vi "Run.vi"(8 "error in (no error)":errorcluster, 11 "socket PUB in":refnum<class "socket PUB.lvclass">) -> (0 "error out":errorcluster, 3 "socket PUB out":refnum<class "socket PUB.lvclass">)   [LabVIEW 2018, in "socket PUB.lvclass"]
uses:
  socket PUB.lvclass
  C:/Users/devstaff/sparc4/s4gui/Versao ZeroMQ REQ-REP/SPARC4_GUI -v1.0.8 - com pacote communication manager/communication-manager/Socket/Socket.lvclass
  State Machine/CM_State Machine.lvclass
  Socket/Socket.lvclass
  RxTx/CM_RxTx.lvclass
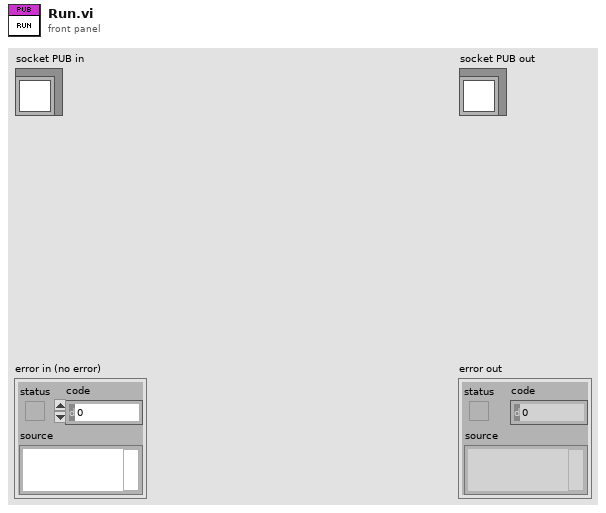
[diagram p1: front panel]
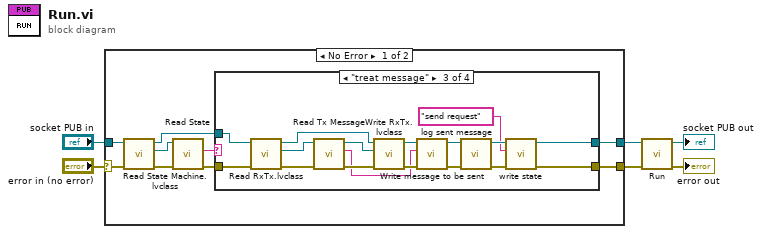
[diagram p0: block diagram]
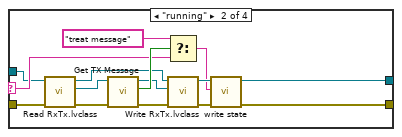
[diagram p3: hidden frame]
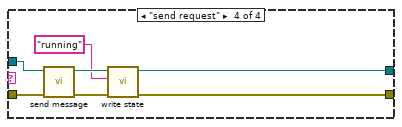
[diagram p4: hidden frame]
diagram:
  n1 = case shown="No Error" "error in (no error)" {
    selector: "error in (no error)" -> [w11 w57]
    tunnel: "socket PUB in" -> [w9 w58]
    tunnel: [w7 w58] -> w4
    tunnel: [w10 w57] -> w1
    frame No Error {
      n2 = call-dynamic "Read State Machine.lvclass.vi"("error in (no error)"=w11, "Socket in"=w9) -> ("error out"=w13:errorcluster, "State Machine.lvclass"=w15:refnum<class "CM_State Machine.lvclass">, "Socket out"=w8:refnum<class "socket PUB.lvclass">)  [unwired: 7 in]
      n3 = call-dynamic "Read State.vi"("error in (no error)"=w13, "State Machine in"=w15) -> ("error out"=w12:errorcluster, "State"=w14:string)  [unwired: 7 in, 1 out]
      n4 = case shown="\"treat message\"" w14 {
        selector: w14 -> [_ w31 _ _]
        tunnel: w8 -> [w17 w24 w42 w56]
        tunnel: [w17 w21 w34 w53] -> w7
        tunnel: [w16 w20 w33 w52] -> w10
        tunnel: w12 -> [w16 w29 w41 w55]
        frame Default {
        }
        frame "running" {
          n5 = call-dynamic "Read RxTx.lvclass.vi"("error in (no error)"=w29, "Socket in"=w24) -> ("error out"=w26:errorcluster, "RxTx.lvclass"=w28:refnum<class "CM_RxTx.lvclass">, "Socket out"=w23:refnum<class "socket PUB.lvclass">)  [unwired: 7 in]
          n6 = call "Get TX Message.vi"("error in (no error)"=w26, "RxTx in"=w28) -> ("error out"=w25:errorcluster, "New msg"=w32:bool, "RxTx out"=w27:refnum<class "CM_RxTx.lvclass">)  [unwired: 7 in]
          n7 = Select(t="treat message", s=w32, f=w31) -> (s? t:f=w18:string)
          n8 = call-dynamic "Write RxTx.lvclass.vi"("error in (no error)"=w25, "RxTx.lvclass"=w27, "Socket in"=w23) -> ("error out"=w19:errorcluster, "Socket out"=w22:refnum<class "socket PUB.lvclass">)  [unwired: 7 in]
          n9 = call "write state.vi"("error in (no error)"=w19, "State"=w18, "Socket in"=w22) -> ("error out"=w20:errorcluster, "Socket out"=w21:refnum<class "socket PUB.lvclass">)  [unwired: 7 in]
        }
        frame "treat message" {
          n10 = call-dynamic "Read RxTx.lvclass.vi"("error in (no error)"=w41, "Socket in"=w42) -> ("error out"=w43:errorcluster, "RxTx.lvclass"=w49:refnum<class "CM_RxTx.lvclass">, "Socket out"=w48:refnum<class "socket PUB.lvclass">)  [unwired: 7 in]
          n11 = call "Read Tx Message.vi"("error in (no error)"=w43, "RxTx in"=w49) -> ("error out"=w45:errorcluster, "Tx Message"=w35:string, "RxTx out"=w44:refnum<class "CM_RxTx.lvclass">)  [unwired: 7 in]
          n12 = call-dynamic "Write RxTx.lvclass.vi"("error in (no error)"=w45, "RxTx.lvclass"=w44, "Socket in"=w48) -> ("error out"=w46:errorcluster, "Socket out"=w47:refnum<class "socket PUB.lvclass">)  [unwired: 7 in]
          n13 = call-dynamic "Write message to be sent.vi"("error in (no error)"=w46, "message to be sent"=w35, "Socket in"=w47) -> ("error out"=w39:errorcluster, "Socket out"=w40:refnum<class "socket PUB.lvclass">)  [unwired: 7 in]
          n14 = call "log sent message.vi"("error in (no error)"=w39, "Socket in"=w40) -> ("error out"=w38:errorcluster, "Socket out"=w37:refnum<class "socket PUB.lvclass">)  [unwired: 8 in]
          n15 = call "write state.vi"("error in (no error)"=w38, "State"="send request" ("new state"), "Socket in"=w37) -> ("error out"=w33:errorcluster, "Socket out"=w34:refnum<class "socket PUB.lvclass">)  [unwired: 7 in]
        }
        frame "send request" {
          n16 = call "send message.vi"("error in (no error)"=w55, "Socket in"=w56) -> ("error out"=w51:errorcluster, "Socket out"=w54:refnum<class "socket PUB.lvclass">)  [unwired: 8 in]
          n17 = call "write state.vi"("error in (no error)"=w51, "State"="running" ("new state"), "Socket in"=w54) -> ("error out"=w52:errorcluster, "Socket out"=w53:refnum<class "socket PUB.lvclass">)  [unwired: 7 in]
        }
      }
    }
    frame Error {
    }
  }
  n18 = call-parent "Run.vi"("error in (no error)"=w1, "Socket in"=w4) -> ("error out"=→"error out":errorcluster, "Socket out"=→"socket PUB out":refnum<class "socket PUB.lvclass">)  [unwired: 8 in]
